vi "Get Slot Parameters.vi"(8 "error in (no error)":errorcluster, 11 "SPECAN_IQSLOT in":refnum<class "SPECAN_IQSLOT.lvclass">) -> (0 "error out":errorcluster, 3 "SPECAN_IQSLOT out":refnum<class "SPECAN_IQSLOT.lvclass">)   [LabVIEW 2018, in "SPECAN_IQSLOT.lvlib" / "SPECAN_IQSLOT.lvclass"]
uses:
  SPECAN_IQSLOT.lvclass
  C:/Sequence Automation/Plugins/Measurement Interface.lvlibp/Measurement Interface.lvclass
  Plugins/Measurement Interface.lvlibp/Private Methods/Measurement Parameters/Read Measurement Parameters.vi
  Plugins/String Database.lvlibp/String Database.lvclass
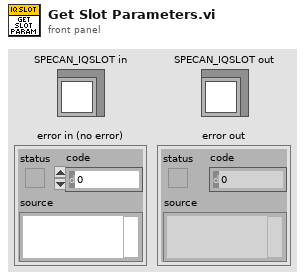
[diagram p1: front panel]
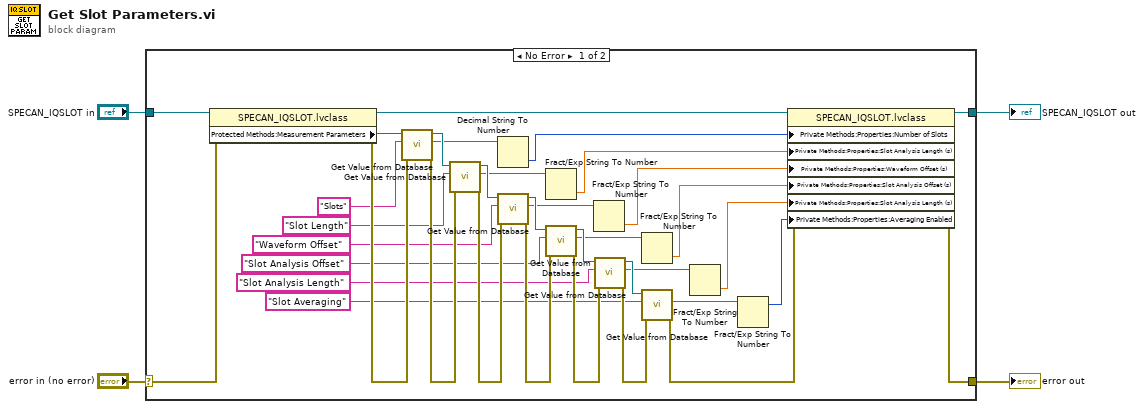
[diagram p0: block diagram]
diagram:
  n1 = case shown="No Error" "error in (no error)" {
    selector: "error in (no error)" -> [w40 w42]
    tunnel: [w36 w42] -> w3
    tunnel: [w35 w41] -> w1
    tunnel: "SPECAN_IQSLOT in" -> [w39 w41]
    frame No Error {
      n2 = property class="SPECAN_IQSLOT.lvclass"(reference=w39, error in=w40) -> (reference out=w5:refnum<class "SPECAN_IQSLOT.lvclass">, error out=w37:errorcluster, "Protected Methods:Measurement Parameters"=w38:refnum<class "String Database.lvclass">)
      n3 = call "Get Value from Database.vi"("error in (no error)"=w37, "Entry Name"="Slots", "Message in"=w38) -> ("error out"=w33:errorcluster, "Entry Value"=w17:string, "Message out"=w34:refnum<class "String Database.lvclass">)  [unwired: 5 in, 1 out]
      n4 = call "Get Value from Database.vi"("error in (no error)"=w33, "Entry Name"="Slot Length", "Message in"=w34) -> ("error out"=w31:errorcluster, "Entry Value"=w13:string, "Message out"=w26:refnum<class "String Database.lvclass">)  [unwired: 5 in, 1 out]
      n5 = Decimal String To Number(string=w17) -> (number=w16:i32)  [unwired: 2 in, 1 out]
      n6 = call "Get Value from Database.vi"("error in (no error)"=w31, "Entry Name"="Waveform Offset", "Message in"=w26) -> ("error out"=w30:errorcluster, "Entry Value"=w12:string, "Message out"=w25:refnum<class "String Database.lvclass">)  [unwired: 5 in, 1 out]
      n7 = Fract/Exp String To Number(string=w13) -> (number=w15:dbl)  [unwired: 3 in, 1 out]
      n8 = call "Get Value from Database.vi"("error in (no error)"=w30, "Entry Name"="Slot Analysis Offset", "Message in"=w25) -> ("error out"=w29:errorcluster, "Entry Value"=w11:string, "Message out"=w24:refnum<class "String Database.lvclass">)  [unwired: 5 in, 1 out]
      n9 = Fract/Exp String To Number(string=w12) -> (number=w6:dbl)  [unwired: 3 in, 1 out]
      n10 = call "Get Value from Database.vi"("error in (no error)"=w29, "Entry Name"="Slot Analysis Length", "Message in"=w24) -> ("error out"=w28:errorcluster, "Entry Value"=w10:string, "Message out"=w23:refnum<class "String Database.lvclass">)  [unwired: 5 in, 1 out]
      n11 = Fract/Exp String To Number(string=w11) -> (number=w7:dbl)  [unwired: 3 in, 1 out]
      n12 = call "Get Value from Database.vi"("error in (no error)"=w28, "Entry Name"="Slot Averaging", "Message in"=w23) -> ("error out"=w27:errorcluster, "Entry Value"=w9:string)  [unwired: 5 in, 2 out]
      n13 = Fract/Exp String To Number(string=w10) -> (number=w8:dbl)  [unwired: 3 in, 1 out]
      n14 = Fract/Exp String To Number(string=w9) -> (offset past number=w14:i32)  [unwired: 3 in, 1 out]
      n15 = property class="SPECAN_IQSLOT.lvclass"(reference=w5, error in=w27, "Private Methods:Properties:Number of Slots"=w16, "Private Methods:Properties:Slot Analysis Length (s)"=w15, "Private Methods:Properties:Waveform Offset (s)"=w6, "Private Methods:Properties:Slot Analysis Offset (s)"=w7, "Private Methods:Properties:Slot Analysis Length (s)"=w8, "Private Methods:Properties:Averaging Enabled"=w14) -> (reference out=w35:refnum<class "SPECAN_IQSLOT.lvclass">, error out=w36:errorcluster)
    }
    frame Error {
    }
  }
  "error out" <- w3
  "SPECAN_IQSLOT out" <- w1
